vi "Do This.vi"(8 "error in (no error)":errorcluster, 10 "Status Events":refnum<class "Status Events.lvclass">, 11 "Job in":refnum<class "Job.lvclass">) -> (0 "error out":errorcluster, 3 "Job out":refnum<class "Job.lvclass">)   [LabVIEW 2014, in "Job.lvclass"]
uses:
  Job.lvclass
  Status Events/Status Events.lvclass
  Job.lvclass/Job.ctl
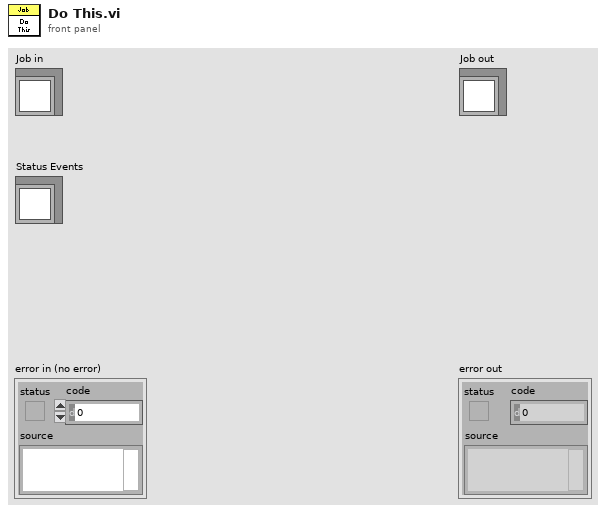
[diagram p1: front panel]
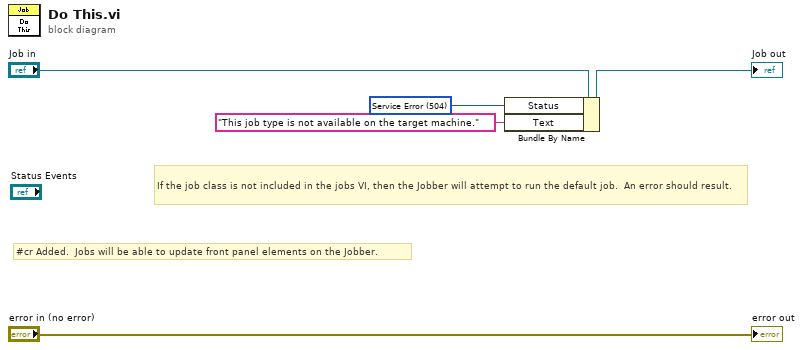
[diagram p0: block diagram]
diagram:
  w3 = u16 504 items=["Service Error"=504, "Abort"=503, "Fail"=500, "Pass"=200] ("Status")
  # "#cr Added.  Jobs will be able to update front panel elements on the Jobber."
  # "If the job class is not included in the jobs VI, then the Jobber will attempt to run the default job.  An error should result."
  n1 = Bundle By Name(cluster="Job in", "Status"=w3, "Text"="This job type is not available on the target machine." ("Results.Text")) -> (→"Job out":refnum<class "Job.lvclass">)
  "error out" <- "error in (no error)"
